vi "GE 5565PIORC.Bit Manipulation.Set Bits (U8).vi"(8 "bit count (1)":i32=1, 9 "bit index":i32, 10 "bits":u8 format="%016x", 11 "packed value in":u8 format="%016x") -> (3 "packed value out":u8 format="%016x")   [LabVIEW 2016, in "GE 5565PIORC.lvclass"]
doc: "This VI extracts a subset of <B>bits</B>, starting with the LSB and up to the length specified by <B>bit count</B>, and overwrites a subset of <B>packed value</B> with these extracted bits starting at <B>bit index</B>."
uses:
  GE 5565PIORC.lvclass
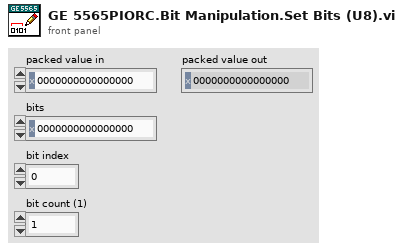
[diagram p1: front panel]
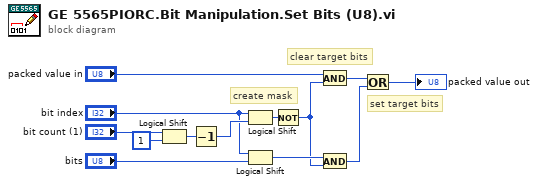
[diagram p0: block diagram]
diagram:
  # "set target bits"
  # "create mask"
  # "clear target bits"
  n1 = Logical Shift(y="bit count (1)", x=u8 1) -> (x << y=w10:u8)
  n2 = Decrement(x=w10) -> (x-1=w9:u8)
  n3 = Logical Shift(y="bit index", x=w9) -> (x << y=w6:u8)
  n4 = Logical Shift(y="bit index", x="bits") -> (x << y=w3:u8)
  n5 = Not(x=w6) -> (.not. x?=w2:u8)
  n6 = And(x="packed value in", y=w2) -> (x .and. y?=w4:u8)
  n7 = And(x=w3, y=w2) -> (x .and. y?=w1:u8)
  n8 = Or(x=w4, y=w1) -> (x .or. y?=→"packed value out":u8)
